vi "RichToFlatniswitch_grpc_RelayControlRequest.vi"(5 "OutputClusterType":T1, 11 "InputCluster":T4) -> (3 "OutputCluster":T1)   [LabVIEW 2021, in "NI Switch_client.lvlib"]
uses:
  NI Switch_client.lvlib
  niswitch_grpc_RelayControlRequest.ctl
  niswitch_grpc_RelayControlRequest_relay_action_enum/niswitch_grpc_RelayControlRequest_relay_action_enum.lvclass
  nidevice_grpc_Session.ctl
  niswitch_grpc_RelayControlRequest_Flat.ctl
  nidevice_grpc_Session_Flat.ctl
  niswitch_grpc_RelayAction.ctl
  niswitch_grpc_RelayControlRequest_relay_action_enum/niswitch_grpc_RelayControlRequest_relay_action_enum.lvclass/niswitch_grpc_RelayControlRequest_relay_action_enum.ctl
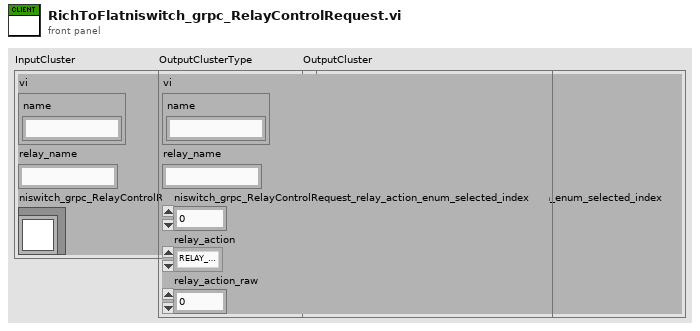
[diagram p1: front panel]
types:
  T1 = typedef "NI Switch_client.lvlib/niswitch_grpc_RelayControlRequest_Flat.ctl" = cluster{"vi":T2, "relay_name":string, "niswitch_grpc_RelayControlRequest_relay_action_enum_selected_index":i32, "relay_action":T3, "relay_action_raw":i32}
  T2 = typedef "NI Switch_client.lvlib/nidevice_grpc_Session_Flat.ctl" = cluster{"name":string}
  T3 = typedef "NI Switch_client.lvlib/niswitch_grpc_RelayAction.ctl" = enum32{"RELAY_ACTION_UNSPECIFIED", "RELAY_ACTION_NISWITCH_VAL_OPEN_RELAY", "RELAY_ACTION_NISWITCH_VAL_CLOSE_RELAY"}
  T4 = typedef "NI Switch_client.lvlib/niswitch_grpc_RelayControlRequest.ctl" = cluster{"vi":T5, "relay_name":string, "niswitch_grpc_RelayControlRequest_relay_action_enum":refnum<class "niswitch_grpc_RelayControlRequest_relay_action_enum.lvclass">}
  T5 = typedef "NI Switch_client.lvlib/nidevice_grpc_Session.ctl" = cluster{"name":string}
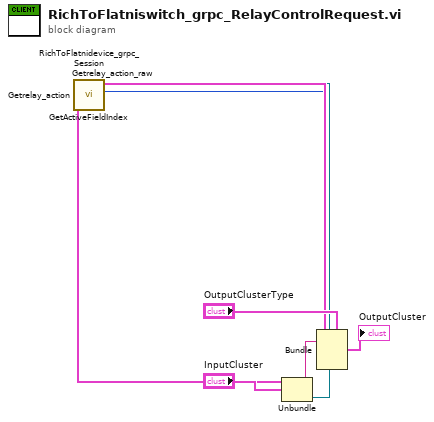
[diagram p0: block diagram]
diagram:
  n1 = Unbundle "Unbundle"("InputCluster") -> ("vi"=w7:T5, "relay_name"=w5:string, "niswitch_grpc_RelayControlRequest_relay_action_enum"=w4:refnum<class "niswitch_grpc_RelayControlRequest_relay_action_enum.lvclass">)
  n2 = call "Getrelay_action_raw.vi"("OneOfTemplate in"=w4) -> ("Get_Val"=w1:i32)  [unwired: 8 in, 2 out]
  n3 = call "Getrelay_action.vi"("OneOfTemplate in"=w4) -> ("Get_Val"=w2:T3)  [unwired: 8 in, 2 out]
  n4 = call "GetActiveFieldIndex.vi"("OneOfTemplate in"=w4) -> ("Active Field Index"=w3:i32)  [unwired: 8 in, 2 out]
  n5 = call "RichToFlatnidevice_grpc_Session.vi"("InputCluster"=w7) -> ("OutputCluster"=w6:T2)  [unwired: 10 in]
  n6 = Bundle "Bundle"(cluster="OutputClusterType", "vi"=w6, "relay_name"=w5, "niswitch_grpc_RelayControlRequest_relay_action_enum_selected_index"=w3, "relay_action"=w2, "relay_action_raw"=w1) -> (→"OutputCluster":T1)
